vi "Voltage Read Array.vi"(8 "error in":errorcluster, 11 "Cycler in":refnum<class "Cycler.lvclass">) -> (0 "error out":errorcluster, 2 "Voltage SP":dbl[](array[numeric]), 3 "Cycler out":refnum<class "Cycler.lvclass">)   [LabVIEW 2023, in "Cycler.lvclass"]
uses:
  Cycler.lvclass
  Cycler.lvclass/Cycler.ctl
  Low Level Capabilities/Voltage/Voltage Setpoint/Voltage Setpoint.lvclass
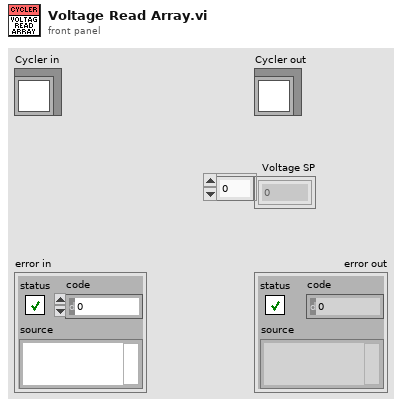
[diagram p1: front panel]
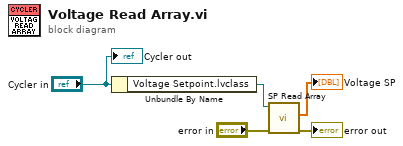
[diagram p0: block diagram]
diagram:
  n1 = Unbundle By Name("Cycler in") -> ("Voltage Setpoint.lvclass"=w2:refnum<class "Voltage Setpoint.lvclass">)
  n2 = call-dynamic "SP Read Array.vi"("error in"="error in", "Voltage Setpoint in"=w2) -> ("error out"=→"error out":errorcluster, "Voltage SP"=→"Voltage SP":dbl[])  [unwired: 6 in, 2 out]
  "Cycler out" <- "Cycler in"
